vi "new_FGGA_Data_Order_Sort.vi"(7 "Data In":string[](array[string])) -> (4 "UDP Data Out":string[](array[string]), 6 "ASCII Ambient(bench)_temp":string, 10 "TCP Data Out":string[](array[string]), 15 "TCP Ambient(bench)_temp":string)   [LabVIEW 2014]
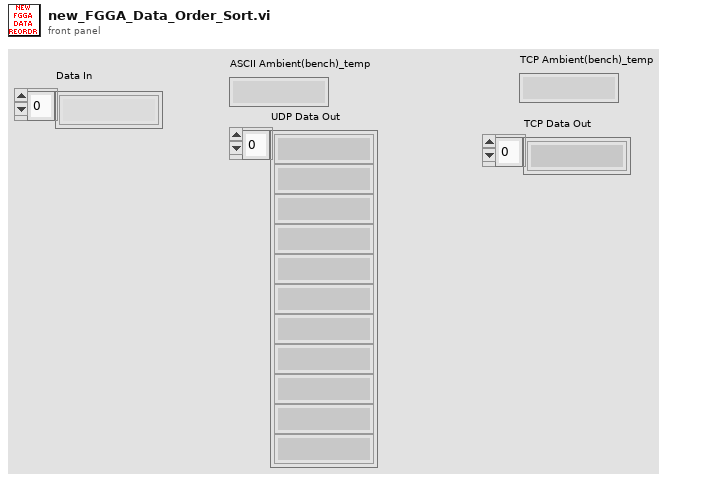
[diagram p1: front panel]
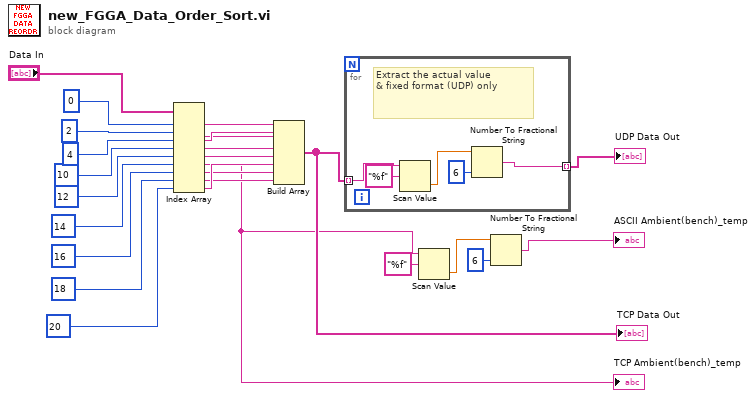
[diagram p0: block diagram]
diagram:
  n1 = Index Array(array="Data In", index #1=0 ("index"), index #2=2 ("index"), index #3=4 ("index"), index #4=10 ("index"), index #5=12 ("index"), index #6=14 ("index"), index #7=16 ("index"), index #8=18 ("index"), index #9=20 ("index")) -> (element #1=w15:string, element #2=w13:string, element #3=w14:string, element #4=w12:string, element #5=w11:string, element #6=w1:string, element #7=w9:string, element #8=w8:string, element #9=w10:string)
  "TCP Ambient(bench)_temp" <- w1
  n2 = Build Array(w15, w14, w13, w12, w11, w10, w9, w8) -> (w2:string[])
  "TCP Data Out" <- w2
  n3 = for {
    tunnel: w2 -> [w29] mode=indexing
    tunnel: [w27] -> w7 mode=indexing
    # "Extract the actual value\n& fixed format (UDP) only"
    n4 = Scan Value(string=w29, format string="%f") -> (value=w26:dbl)  [unwired: 1 in, 1 out]
    n5 = Number To Fractional String(number=w26, precision (6)=i16 6) -> (F-format string=w27:string)  [unwired: 2 in]
  }
  "UDP Data Out" <- w7
  n6 = Scan Value(string=w1, format string="%f") -> (value=w4:dbl)  [unwired: 1 in, 1 out]
  n7 = Number To Fractional String(number=w4, precision (6)=i16 6) -> (F-format string=→"ASCII Ambient(bench)_temp":string)  [unwired: 2 in]
